vi "tcs_putSample_kernelDawdleFilter.vi"(8 "error in (no error)":errorcluster, 11 "kernel_DawdleFilter_Ctl":T1) -> (0 "error out":errorcluster, 2 "function return":i32, 3 "kernel_DawdleFilter_Ctl out":T1)   [LabVIEW 2016, in "SALLV_tcs.lvlib"]
doc: "int tcs_shm_putSample_kernel_DawdleFilterLV(tcs_kernel_DawdleFilterLV *kernel_DawdleFilter_Ctl );"
uses:
  SALLV_tcs.lvlib
  DataTypes/kernel_DawdleFilter.ctl
  SALLV_tcs.so
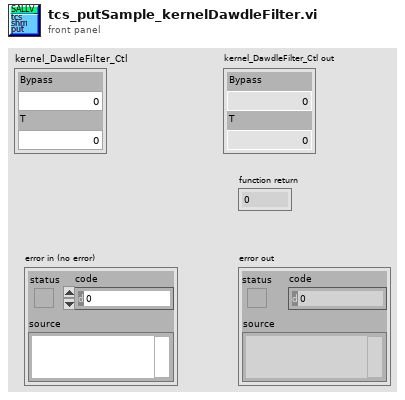
[diagram p1: front panel]
types:
  T1 = typedef "SALLV_tcs.lvlib/kernel_DawdleFilter.ctl" = cluster{"Bypass":i32, "T":sgl}
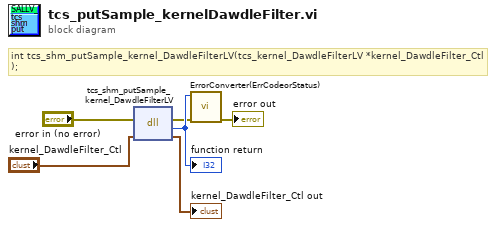
[diagram p0: block diagram]
diagram:
  # "int tcs_shm_putSample_kernel_DawdleFilterLV(tcs_kernel_DawdleFilterLV *kernel_DawdleFilter_Ctl );"
  n1 = dll-call lib="home/andres/Desktop/SALLV_tcs/SALLV_tcs.*" fn="tcs_shm_putSample_kernel_DawdleFilterLV"(error in="error in (no error)", "kernel_DawdleFilter_Ctl"="kernel_DawdleFilter_Ctl") -> (error out=w2:errorcluster, w6:i32, "kernel_DawdleFilter_Ctl"=→"kernel_DawdleFilter_Ctl out":T1)  [unwired: 2 in, 1 out]
  "function return" <- w6
  n2 = call "ErrorConverter(ErrCodeorStatus).vi"("error in (no error)"=w2, "error code"=w6) -> ("error out"=→"error out":errorcluster)  [unwired: 9 in]
